vi "Initialize-parameter-refs.vi"(8 "error in (no error)":errorcluster, 10 "VI ref":refnum<vi>, 11 "UI ref. in":refnum<data-value>) -> (0 "error out":errorcluster, 3 "UI ref.":refnum<data-value>)   [LabVIEW 2013, in "CameraVision.lvlib" / "CV-UI.lvclass"]
uses:
  CV-UI.lvclass
  Parameter-group-names.ctl
  CV-UI.lvclass/CV-UI.ctl
panel:
  in  "Parameter refs":T1
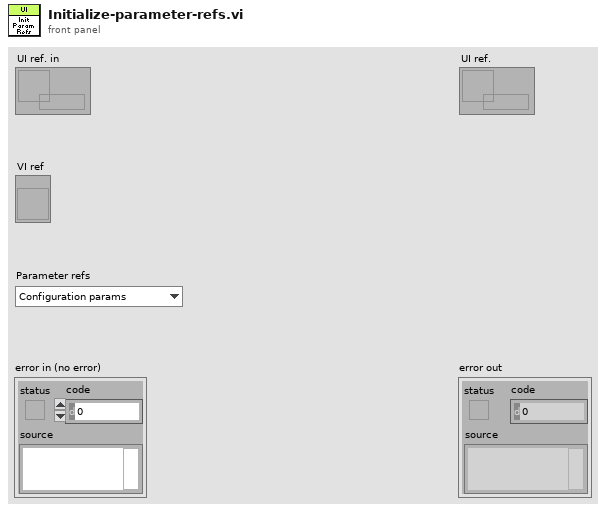
[diagram p1: front panel]
types:
  T1 = typedef "CameraVision.lvlib/CV-UI.lvclass/Parameter-group-names.ctl" = enum16{"Configuration params", "Acquisition params", "Correction params", "Analysis params", "Temperature params", "Mapping params", "Storage params", "Filter params"}
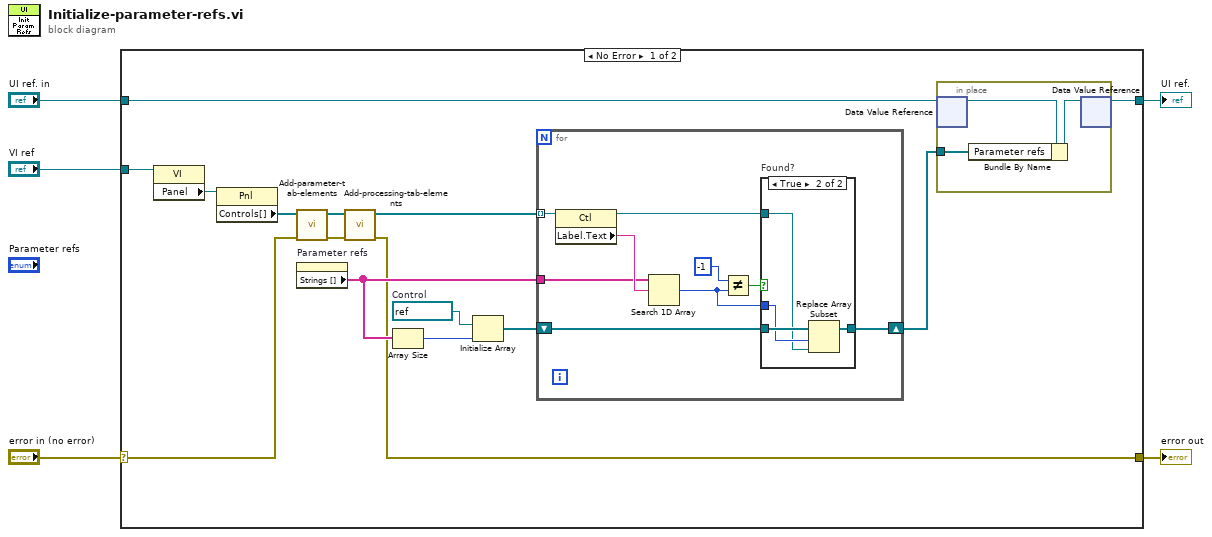
[diagram p0: block diagram]
diagram:
  n1 = case shown="No Error" "error in (no error)" {
    selector: "error in (no error)" -> [w15 w39]
    tunnel: [w9 w39] -> w4
    tunnel: [w7 w38] -> w2
    tunnel: "UI ref. in" -> [w8 w38]
    tunnel: "VI ref" -> [w20 _]
    frame No Error {
      w11 = refnum<vi> refnum  # Control
      n2 = property class="VI"(reference=w20) -> ("Panel"=w19:refnum<vi>)  [unwired: 1 in, 2 out]
      n3 = property class="Pnl"(reference=w19) -> ("Controls[]"=w18:refnum<vi>[])  [unwired: 1 in, 2 out]
      n4 = call "Add-parameter-tab-elements.vi"("error in (no error)"=w15, "Controls in"=w18) -> ("error out"=w16:errorcluster, "Controls out"=w17:refnum<vi>[])  [unwired: 8 in]
      n5 = property on="Parameter refs" class="Enum (strict)"() -> ("Strings []"=w12:string[])  [unwired: 2 in, 2 out]
      n6 = call "Add-processing-tab-elements.vi"("error in (no error)"=w16, "Controls in"=w17) -> ("error out"=w9:errorcluster, "Controls out"=w10:refnum<vi>[])  [unwired: 8 in]
      n7 = Array Size(array=w12) -> (size(s)=w14:i32)
      n8 = Initialize Array(w11, w14) -> (w13:refnum<vi>[])
      n9 = for {
        tunnel: w10 -> [w32] mode=indexing
        tunnel: w12 -> [w30]
        shift-right: [w27] -> w6
        shift-left: w13 -> [w28]
        n10 = property class="Ctl"(reference=w32) -> (reference out=w26:refnum<vi>, "Label.Text"=w31:string)  [unwired: 1 in, 1 out]
        n11 = Search 1D Array(1D array=w30, element=w31) -> (index of element=w25:i32)  [unwired: 1 in]
        n12 = Not Equal?(x=-1, y=w25) -> (x != y?=w24:bool)
        n13 = case "Found?" shown="True" w24 {
          tunnel: w28 -> [w33 w37]
          tunnel: [w33 w36] -> w27
          tunnel: w26 -> [_ w34]
          tunnel: w25 -> [_ w35]
          frame False {
          }
          frame True {
            n14 = Replace Array Subset(array=w37, new element=w34, index=w35) -> (w36:refnum<vi>[])
          }
        }
      }
      n15 = in-place {
        in-place-border: w6 -> [w21]
        n16 = in-place-dvr #1(w8) -> (w23:refnum<class "CV-UI.lvclass">)  [unwired: 1 out]
        n17 = Bundle By Name(cluster=w23, "Parameter refs"=w21) -> (w22:refnum<class "CV-UI.lvclass">)
        n18 = in-place-dvr #1(w22) -> (w7:refnum<data-value>)  [unwired: 1 out]
      }
    }
    frame Error {
    }
  }
  "error out" <- w4
  "UI ref." <- w2
